vi "atcs_monitorCommand_Offset.vi"(8 "error in (no error)":errorcluster, 11 "command_Offset_Ctl":T1) -> (0 "error out":errorcluster, 2 "function return":i32, 3 "command_Offset_Ctl out":T1)   [LabVIEW 2016, in "SALLV_atcs.lvlib"]
doc: "int atcs_shm_monitorCommand_OffsetLV(atcs_command_OffsetLV *command_Offset_Ctl );"
uses:
  SALLV_atcs.lvlib
  DataTypes/command_Offset.ctl
  SALLV_atcs.so
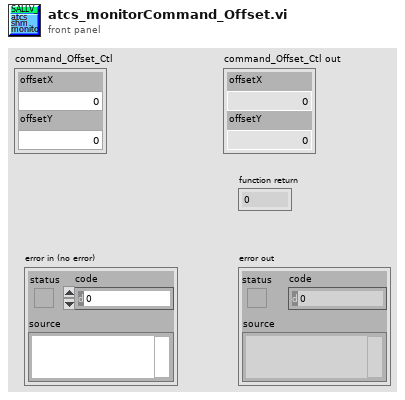
[diagram p1: front panel]
types:
  T1 = typedef "SALLV_atcs.lvlib/command_Offset.ctl" = cluster{"offsetX":dbl, "offsetY":dbl}
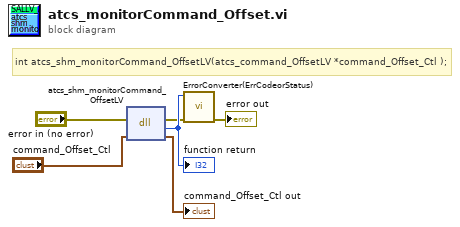
[diagram p0: block diagram]
diagram:
  # "int atcs_shm_monitorCommand_OffsetLV(atcs_command_OffsetLV *command_Offset_Ctl );"
  n1 = dll-call lib="home/andres/Desktop/SALLV_atcs/SALLV_atcs.*" fn="atcs_shm_monitorCommand_OffsetLV"(error in="error in (no error)", "command_Offset_Ctl"="command_Offset_Ctl") -> (error out=w2:errorcluster, w6:i32, "command_Offset_Ctl"=→"command_Offset_Ctl out":T1)  [unwired: 2 in, 1 out]
  "function return" <- w6
  n2 = call "ErrorConverter(ErrCodeorStatus).vi"("error in (no error)"=w2, "error code"=w6) -> ("error out"=→"error out":errorcluster)  [unwired: 9 in]
